vi "Test A.vi"(1 "board image":T1) -> (0 "Pass?":T2)   [LabVIEW 2023]
doc: "Test a basic DAQ board image."
uses:
  Common/Pass Fail Boolean.ctl
  Common/Board Image.ctl
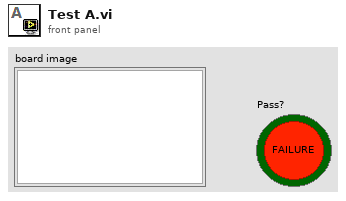
[diagram p1: front panel]
types:
  T1 = typedef "Board Image.ctl" = picture
  T2 = typedef "Pass Fail Boolean.ctl" = bool
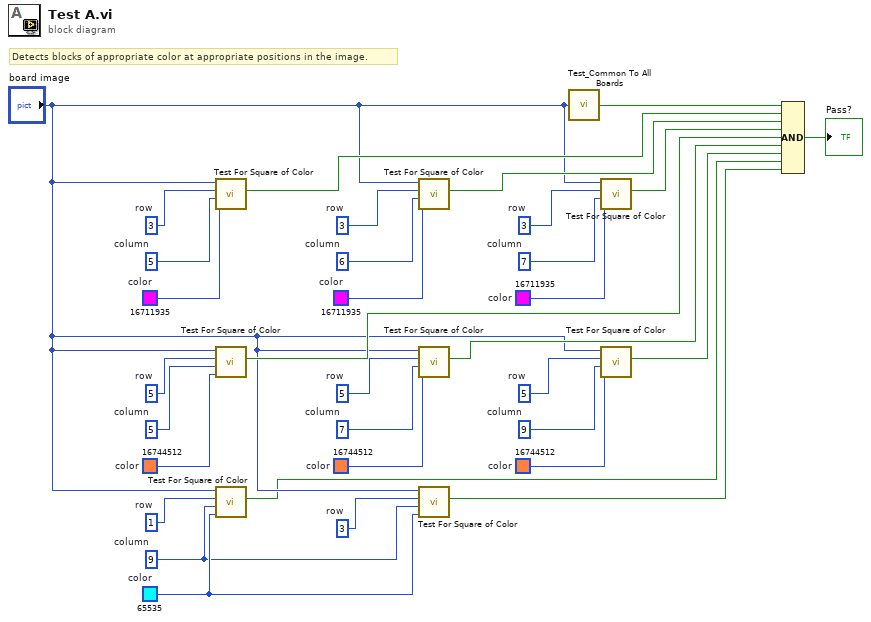
[diagram p0: block diagram]
diagram:
  w2 = u32 65535  # color
  w12 = i16 9  # column
  w11 = i16 5  # row
  w13 = u32 16744512  # color
  w15 = i16 7  # column
  w16 = i16 5  # row
  w14 = u32 16744512  # color
  w18 = i16 5  # column
  w17 = i16 5  # row
  w19 = u32 16744512  # color
  w30 = i16 7  # column
  w31 = i16 3  # row
  w29 = u32 16711935  # color
  w27 = i16 6  # column
  w26 = i16 3  # row
  w28 = u32 16711935  # color
  w24 = i16 5  # column
  w25 = i16 3  # row
  w23 = u32 16711935  # color
  w33 = i16 3  # row
  w1 = i16 9  # column
  w3 = i16 1  # row
  # "Detects blocks of appropriate color at appropriate positions in the image."
  n1 = call "Test For Square of Color.vi"("color"=w23, "column"=w24, "row"=w25, "board image"="board image") -> ("pass?"=w22:T2)  [unwired: 7 in]
  n2 = call "Test For Square of Color.vi"("color"=w19, "column"=w18, "row"=w17, "board image"="board image") -> ("pass?"=w10:T2)  [unwired: 7 in]
  n3 = call "Test For Square of Color.vi"("color"=w2, "column"=w1, "row"=w3, "board image"="board image") -> ("pass?"=w5:T2)  [unwired: 7 in]
  n4 = call "Test For Square of Color.vi"("color"=w28, "column"=w27, "row"=w26, "board image"="board image") -> ("pass?"=w21:T2)  [unwired: 7 in]
  n5 = call "Test For Square of Color.vi"("color"=w14, "column"=w15, "row"=w16, "board image"="board image") -> ("pass?"=w9:T2)  [unwired: 7 in]
  n6 = call "Test For Square of Color.vi"("color"=w2, "column"=w1, "row"=w33, "board image"="board image") -> ("pass?"=w4:T2)  [unwired: 7 in]
  n7 = call "Test_Common To All Boards.vi"("board image"="board image") -> ("pass?"=w7:T2)
  n8 = call "Test For Square of Color.vi"("color"=w29, "column"=w30, "row"=w31, "board image"="board image") -> ("pass?"=w20:T2)  [unwired: 7 in]
  n9 = call "Test For Square of Color.vi"("color"=w13, "column"=w12, "row"=w11, "board image"="board image") -> ("pass?"=w8:T2)  [unwired: 7 in]
  n10 = Compound Arithmetic op=AND(w7, w22, w21, w20, w10, w9, w8, w5, w4) -> (→"Pass?":T2)
